vi "DSF.Engine.Plugin.Rx.vi"(8 "error in (no error)":errorcluster, 10 "Transfer Group in":refnum<class "DSF.Engine.Transfer Group.lvclass">, 11 "Plugin in":refnum<class "DSF.Engine.Plugin.lvclass">) -> (0 "error out":errorcluster, 2 "Transfer Group out":refnum<class "DSF.Engine.Transfer Group.lvclass">, 3 "Plugin out":refnum<class "DSF.Engine.Plugin.lvclass">)   [LabVIEW 2017, in "DSF.Engine.lvlib" / "DSF.Engine.Plugin.lvclass"]
uses:
  DSF.Engine.Plugin.lvclass
  Transfer/DSF.Engine.Transfer Group.lvclass
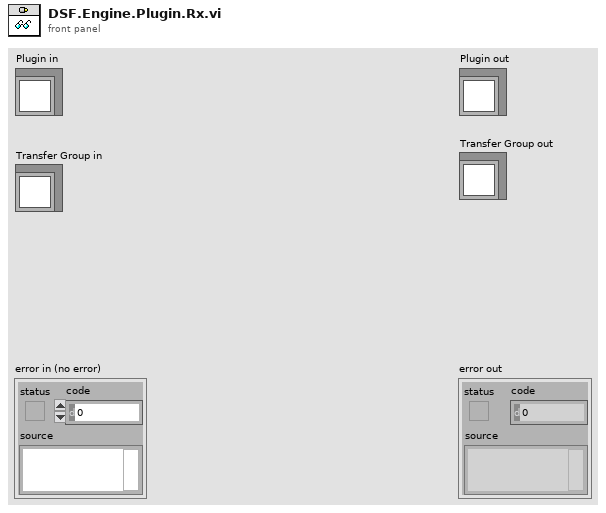
[diagram p1: front panel]
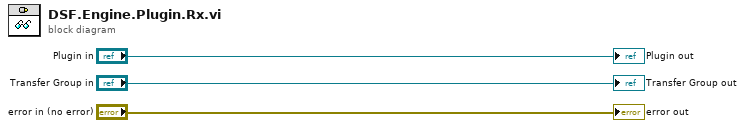
[diagram p0: block diagram]
diagram:
  "error out" <- "error in (no error)"
  "Plugin out" <- "Plugin in"
  "Transfer Group out" <- "Transfer Group in"
